vi "zlib Path.vi"(8 "error in (no error)":errorcluster) -> (0 "error out":errorcluster, 2 "Exists?":bool, 3 "zlib.dll Path":path)   [LabVIEW 2021, in "VI-Hacker.lvlib"]
uses:
  VI-Hacker.lvlib
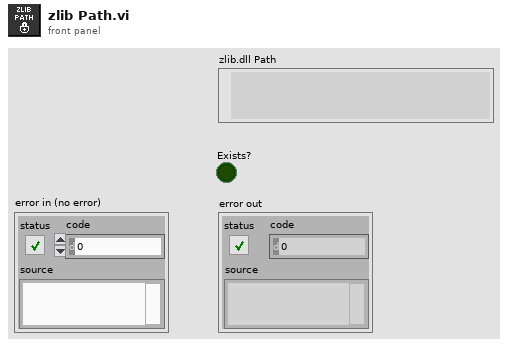
[diagram p1: front panel]
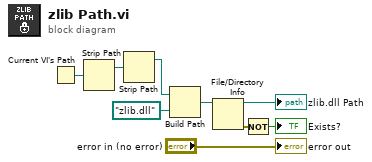
[diagram p0: block diagram]
diagram:
  n1 = Current VI's Path() -> (path=w8:path)
  n2 = Strip Path(path=w8) -> (stripped path=w7:path)  [unwired: 1 out]
  n3 = Strip Path(path=w7) -> (stripped path=w5:path)  [unwired: 1 out]
  n4 = Build Path(base path=w5, name or relative path=path "zlib.dll") -> (appended path=w6:path)
  n5 = File/Directory Info(path=w6) -> (path out=→"zlib.dll Path":path, error out=w2:errorcluster)  [unwired: 1 in, 5 out]
  n6 = Not(x=w2) -> (.not. x?=→"Exists?":bool)
  "error out" <- "error in (no error)"
